vi "L08.vi"() -> ()   [LabVIEW 2012]
panel:
  out "Array":i64[](array[numeric])
  out "string":string
  out "Waveform Graph":i64[](graph)
  out "max":i64
  out "byte array":u8[](array[numeric])
  # "2972712960"
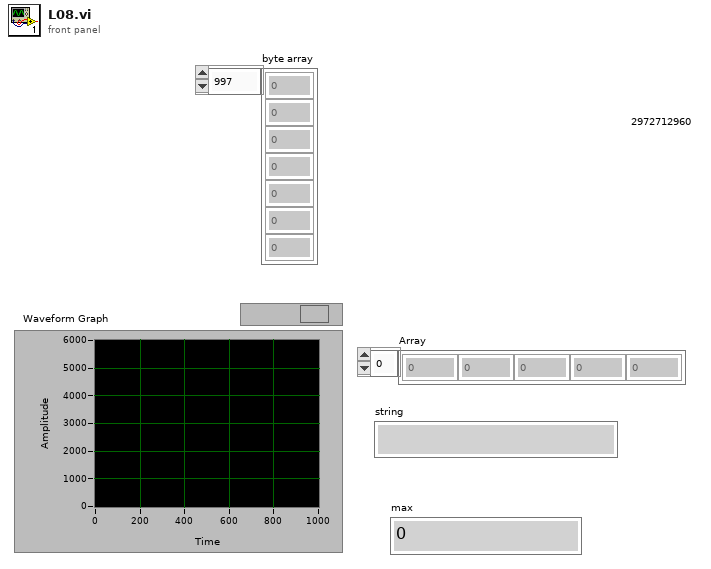
[diagram p1: front panel]
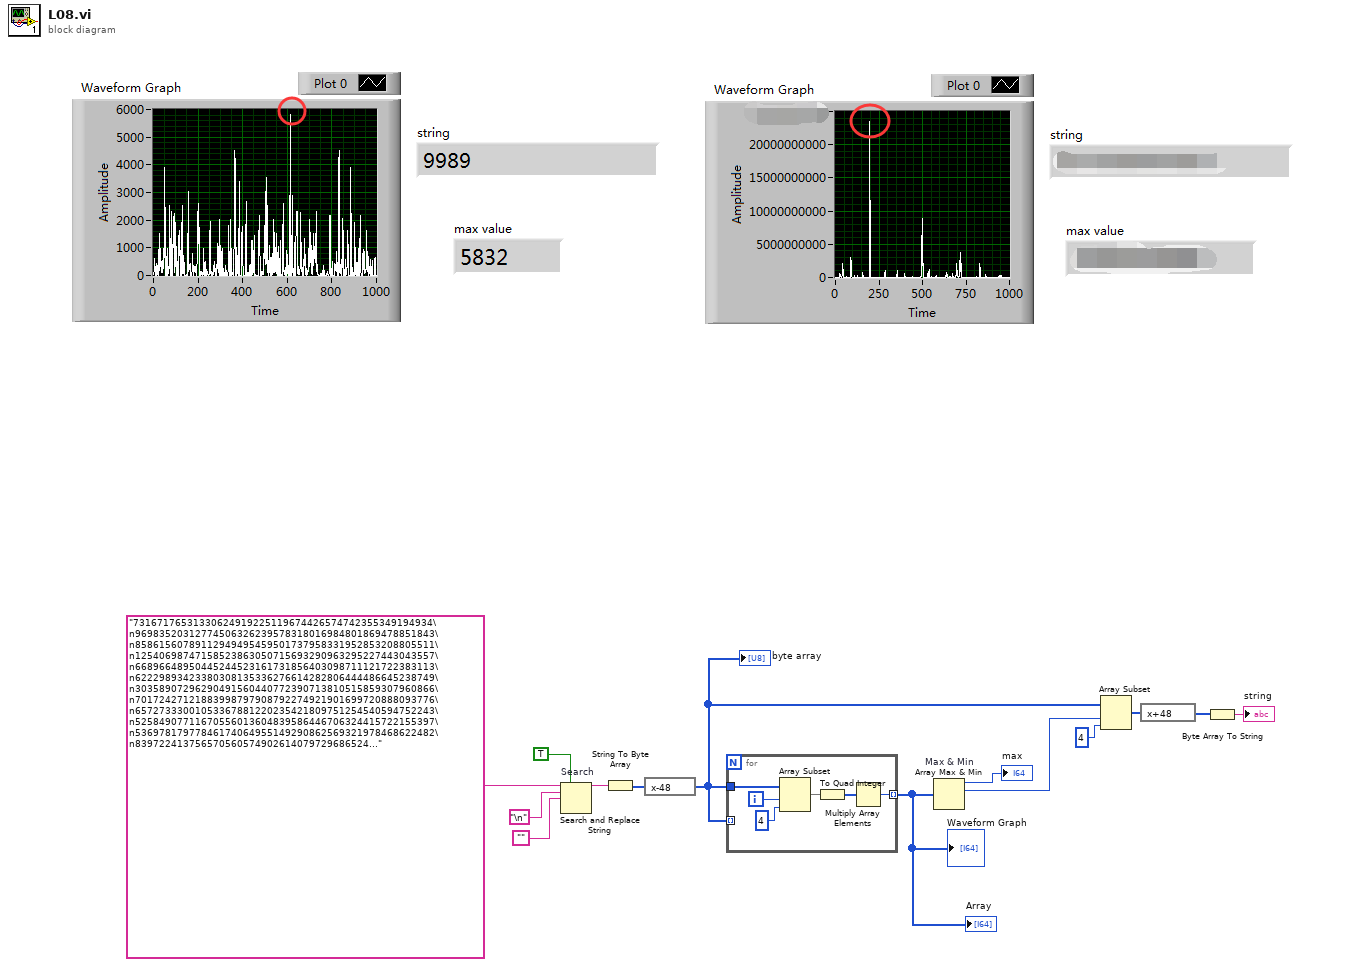
[diagram p0: block diagram]
diagram:
  n1 = Search and Replace String "Search"(replace all?=TRUE ("replace all? (F)"), input string="73167176531330624919225119674426574742355349194934\n96983520312774506326239578318016984801869478851843\n85861560789112949495459501737958331952853208805511\n12540698747158523863050715693290963295227443043557\n66896648950445244523161731856403098711121722383113\n62229893423380308135336276614282806444486645238749\n30358907296290491560440772390713810515859307960866\n70172427121883998797908792274921901699720888093776\n65727333001053367881220235421809751254540594752243\n52584907711670556013604839586446706324415722155397\n53697817977846174064955149290862569321978468622482\n83972241375657056057490261407972968652414535100474\n82166370484403199890008895243450658541227588666881\n16427171479924442928230863465674813919123162824586\n17866458359124566529476545682848912883142607690042\n24219022671055626321111109370544217506941658960408\n07198403850962455444362981230987879927244284909188\n84580156166097919133875499200524063689912560717606\n05886116467109405077541002256983155200055935729725\n71636269561882670428252483600823257530420752963450", search string="\n", replace string="") -> (result string=w12:string)  [unwired: 4 in, 3 out]
  n2 = String To Byte Array(string=w12) -> (unsigned byte array=w11:u8[])
  n3 = expression code="x-48"(w11) -> (w7:u8[])
  "byte array" <- w7
  n4 = for {
    tunnel: w7 -> [w20]
    tunnel: w7 -> [_] mode=indexing
    tunnel: [w17] -> w4 mode=indexing
    i -> [w19]
    n5 = Array Subset "Array Subset"(array=w20, index=w19, length=4) -> (w16:u8[])
    n6 = To Quad Integer(1:w16) -> (0:w15:i64[])
    n7 = Multiply Array Elements(1:w15) -> (0:w17:i64)
  }
  "Waveform Graph" <- w4
  "Array" <- w4
  n8 = Array Max & Min "Max & Min"(array=w4) -> (max value=→"max":i64, max index (indices)=w6:i32)  [unwired: 2 out]
  n9 = Array Subset "Array Subset"(array=w7, index=w6, length=4) -> (w3:u8[])
  n10 = expression code="x+48"(w3) -> (w2:u8[])
  n11 = Byte Array To String(unsigned byte array=w2) -> (string=→"string":string)
